vi "CAN_init.vi"(0 "Control Mode":T2=enum."Position", 5 "error in":errorcluster, 6 "P":dbl=100.0, 7 "P Speed":dbl=1.0, 8 "I":dbl=0.1, 9 "I Speed":dbl=0.01, 10 "D":dbl, 11 "D Speed":dbl) -> (14 "output cluster":T4, 19 "error out":errorcluster)   [LabVIEW 2009, in "OWNCAN.lvlib"]
uses:
  OWNCAN.lvlib
  CAN/SubVIs/CAN Jaguar Control Mode.ctl
  CAN/SubVIs/CAN Jaguar Ref.ctl
  CAN/SubVIs/CAN Jaguar Position Reference.ctl
  Serial.lvlib
  CAN.lvlib
panel:
  in  "Maximum Output Voltage":dbl=5.0
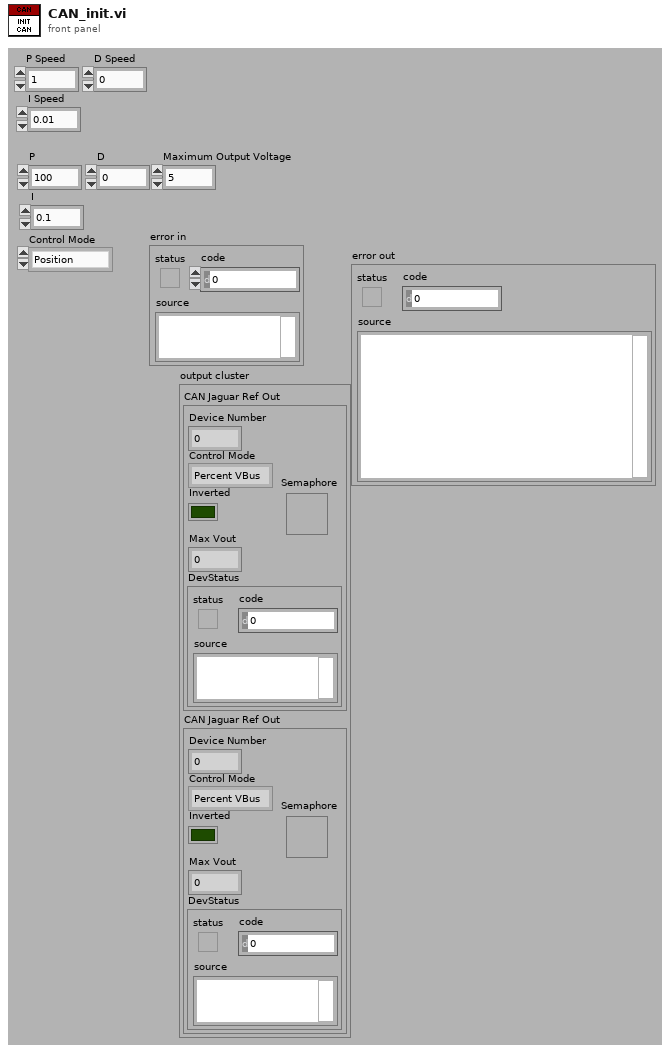
[diagram p1: front panel]
types:
  T1 = typedef "CAN.lvlib/CAN Jaguar Ref.ctl" = cluster{"Device Number":u8, "Control Mode":T2, "Inverted":bool, "Semaphore":T3, "Max Vout":dbl, "DevStatus":errorcluster}
  T2 = typedef "CAN.lvlib/CAN Jaguar Control Mode.ctl" = enum16{"Percent VBus", "Speed", "Position", "Current"}
  T3 = typedef "Semaphore RefNum" = refnum<k1>
  T4 = cluster{"CAN Jaguar Ref Out":T1, "CAN Jaguar Ref Out":T1}
  T5 = typedef "CAN.lvlib/CAN Jaguar Position Reference.ctl" = enum16{"Encoder", "Potentiometer"}
  T6 = cluster{"P Speed":dbl, "I Speed":dbl, "D Speed":dbl}
  T7 = cluster{cluster{"P":dbl, "I":dbl, "D":dbl}, cluster{"P Speed":dbl, "I Speed":dbl, "D Speed":dbl}}
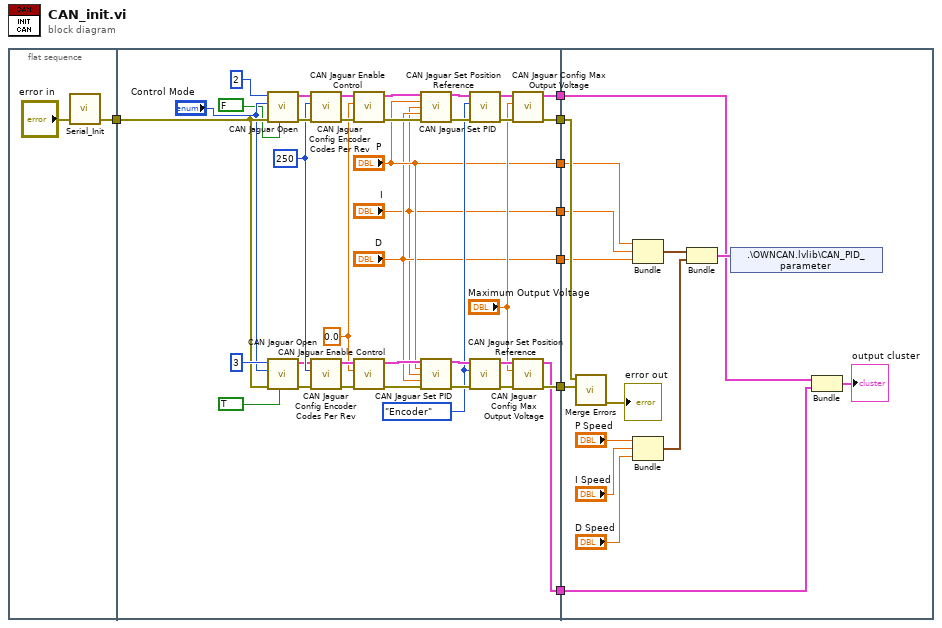
[diagram p0: block diagram]
diagram:
  n1 = flat-sequence {
    tunnel: [w9] -> w8
    tunnel: w8 -> [w21]
    tunnel: [w19] -> w7
    tunnel: [w18] -> w6
    tunnel: [w17] -> w5
    tunnel: [w16] -> w4
    tunnel: ["P"] -> w3
    tunnel: ["I"] -> w2
    tunnel: ["D"] -> w1
    tunnel: w7 -> [w62]
    tunnel: w6 -> [w61]
    tunnel: w5 -> [w49]
    tunnel: w4 -> [w50]
    tunnel: w3 -> [w56]
    tunnel: w2 -> [w55]
    tunnel: w1 -> [w54]
    frame #0 {
      n2 = call "Serial_Init.vi"("error in (no error)"="error in") -> ("error out"=w9:errorcluster)  [unwired: 3 in, 1 out]
    }
    frame #1 {
      w27 = 0.0 ("Encoder Initial Position")
      w28 = CAN_Jaguar_Position_Reference."Encoder" ("Position Reference")
      w43 = u16 250 ("Encoder Codes Per Rev")
      n3 = call "CAN Jaguar Open.vi"("Inverted"=FALSE, "error in (no error)"=w21, "Control Mode"="Control Mode", "Device Number"=u8 2) -> ("error out"=w44:errorcluster, "CAN Jaguar Ref Out"=w41:T1)  [unwired: 6 in]
      n4 = call "CAN Jaguar Open.vi"("Inverted"=TRUE, "error in (no error)"=w21, "Control Mode"="Control Mode", "Device Number"=u8 3) -> ("error out"=w45:errorcluster, "CAN Jaguar Ref Out"=w42:T1)  [unwired: 6 in]
      n5 = call "CAN Jaguar Config Encoder Codes Per Rev.vi"("error in (no error)"=w44, "Encoder Codes Per Rev"=w43, "CAN Jaguar Ref"=w41) -> ("error out"=w38:errorcluster, "CAN Jaguar Ref Out"=w37:T1)  [unwired: 7 in]
      n6 = call "CAN Jaguar Config Encoder Codes Per Rev.vi"("error in (no error)"=w45, "Encoder Codes Per Rev"=w43, "CAN Jaguar Ref"=w42) -> ("error out"=w40:errorcluster, "CAN Jaguar Ref Out"=w39:T1)  [unwired: 7 in]
      n7 = call "CAN Jaguar Enable Control.vi"("error in (no error)"=w38, "Encoder Initial Position"=w27, "CAN Jaguar Ref"=w37) -> ("error out"=w34:errorcluster, "CAN Jaguar Ref Out"=w36:T1)  [unwired: 7 in]
      n8 = call "CAN Jaguar Enable Control.vi"("error in (no error)"=w40, "Encoder Initial Position"=w27, "CAN Jaguar Ref"=w39) -> ("error out"=w33:errorcluster, "CAN Jaguar Ref Out"=w35:T1)  [unwired: 7 in]
      n9 = call "CAN Jaguar Set PID.vi"("CAN Jaguar Ref"=w36, "P"="P", "I"="I", "D"="D", "error in (no error)"=w34) -> ("CAN Jaguar Ref Out"=w32:T1, "error out"=w31:errorcluster)  [unwired: 9 in]
      n10 = call "CAN Jaguar Set PID.vi"("CAN Jaguar Ref"=w35, "P"="P", "I"="I", "D"="D", "error in (no error)"=w33) -> ("CAN Jaguar Ref Out"=w30:T1, "error out"=w29:errorcluster)  [unwired: 9 in]
      n11 = call "CAN Jaguar Set Position Reference.vi"("error in (no error)"=w31, "Position Reference"=w28, "CAN Jaguar Ref"=w32) -> ("error out"=w24:errorcluster, "CAN Jaguar Ref Out"=w25:T1)  [unwired: 7 in]
      n12 = call "CAN Jaguar Set Position Reference.vi"("error in (no error)"=w29, "Position Reference"=w28, "CAN Jaguar Ref"=w30) -> ("error out"=w23:errorcluster, "CAN Jaguar Ref Out"=w26:T1)  [unwired: 7 in]
      n13 = call "CAN Jaguar Config Max Output Voltage.vi"("error in (no error)"=w24, "Maximum Output Voltage"="Maximum Output Voltage", "CAN Jaguar Ref"=w25) -> ("error out"=w18:errorcluster, "CAN Jaguar Ref Out"=w16:T1)  [unwired: 7 in]
      n14 = call "CAN Jaguar Config Max Output Voltage.vi"("error in (no error)"=w23, "Maximum Output Voltage"="Maximum Output Voltage", "CAN Jaguar Ref"=w26) -> ("error out"=w19:errorcluster, "CAN Jaguar Ref Out"=w17:T1)  [unwired: 7 in]
    }
    frame #2 {
      n15 = call <vilib>:"Merge Errors.vi"("error in 2 (no error)"=w62, "error in 1 (no error)"=w61) -> ("error out"=→"error out":errorcluster)  [unwired: 5 in]
      n16 = Bundle ("Position PID")("P"=w56, "I"=w55, "D"=w54) -> (w52:cluster{"P":dbl, "I":dbl, "D":dbl})  [unwired: 1 in]
      n17 = Bundle ("Speed PID")("P Speed"="P Speed", "I Speed"="I Speed", "D Speed"="D Speed") -> (w53:T6)  [unwired: 1 in]
      n18 = Bundle ("PID Parameters\nPID Parameters")(w52, w53) -> (w51:T7)  [unwired: 1 in]
      n19 = shared-variable ".\\OWNCAN.lvlib\\CAN_PID_parameter"(w51) -> ()  [unwired: 1 in, 1 out]
      n20 = Bundle("CAN Jaguar Ref Out"=w50, "CAN Jaguar Ref Out"=w49) -> (→"output cluster":T4)  [unwired: 1 in]
    }
  }
